vi "templates make field PI.vi"(9 "Field Information  2":T1) -> (1 "Field Information":T1)   [LabVIEW 2011]
uses:
  server/database/Fields/Field Record.ctl
  server/database/Fields/Field DataTypes.ctl
  server/database/Fields/Field NextItem.ctl
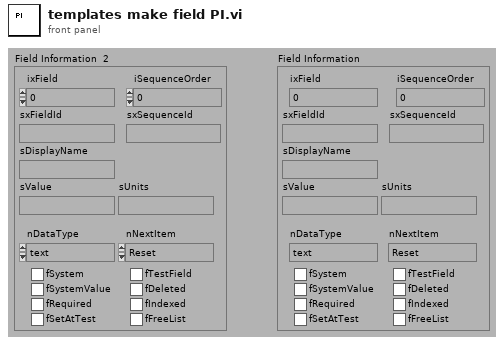
[diagram p1: front panel]
types:
  T1 = typedef "Field Record.ctl" = cluster{"ixField":i32, "iSequenceOrder":i32, "sxFieldId":string, "sxSequenceId":string, "sDisplayName":string, "sValue":string, "sUnits":string, "nDataType":T2, "nNextItem":T3, "fSystem":bool, "fSystemValue":bool, "fRequired":bool, "fSetAtTest":bool, "fTestField":bool, "fDeleted":bool, "fIndexed":bool, "fFreeList":bool}
  T2 = typedef "Field DataTypes.ctl" = enum32{"text", "numeric", "list", "timestamp", "boolean"}
  T3 = typedef "Field NextItem.ctl" = enum32{"Reset", "Retain", "Auto-Increment"}
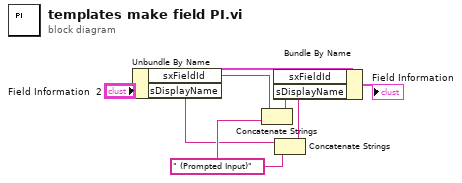
[diagram p0: block diagram]
diagram:
  w5 = " (Prompted Input)"
  n1 = Unbundle By Name("Field Information  2") -> ("sxFieldId"=w6:string, "sDisplayName"=w3:string)
  n2 = Concatenate Strings(w6, w5) -> (w7:string)
  n3 = Concatenate Strings(w3, w5) -> (w4:string)
  n4 = Bundle By Name(cluster="Field Information  2", "sxFieldId"=w7, "sDisplayName"=w4) -> (→"Field Information":T1)
